vi "Number Count Down.vi"   [LabVIEW 2017]
doc: "Polymorphic wrapper that counts a number down once per call, for a single value or for every element of an array."
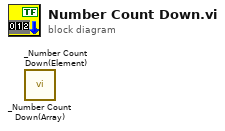
[diagram p0: block diagram]
diagram:
  n1 = call "_Number Count Down(Array).vi"() -> ()  [unwired: 8 in, 2 out]
  n2 = call "_Number Count Down(Element).vi"() -> ()  [unwired: 8 in, 2 out]
